vi "Create Asset.vi"(4 "Asset Class":enum16{"Undefined", "Asset", "Dut", "Fixture"}(ring), 5 "Vendor Number":u32, 6 "Bus Type":T1(ring), 7 "Vendor Name":string, 8 "Error In":errorcluster, 9 "Serial Number":string, 10 "Model Number":u32, 11 "Model Name":string) -> (0 "Error Out":errorcluster, 3 "Asset":refnum<class "Asset.lvclass">)   [LabVIEW 2019, in "Asset.lvclass"]
doc: "Creates an asset based on the properties that uniquely identify it."
uses:
  Asset.lvclass
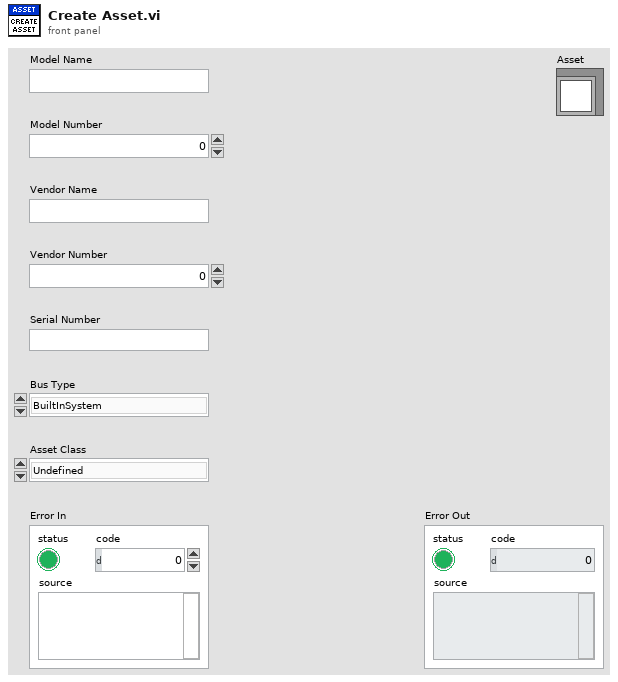
[diagram p1: front panel]
types:
  T1 = enum16{"BuiltInSystem", "PciPxi", "Usb", "Gpib", "Vxi", "Serial", "TcpIp", "cRio", "Scxi", "cDaq", "SwitchBlock", "Scc", "FireWire", "Accessory", "Can", "SwitchBlockDevice"}
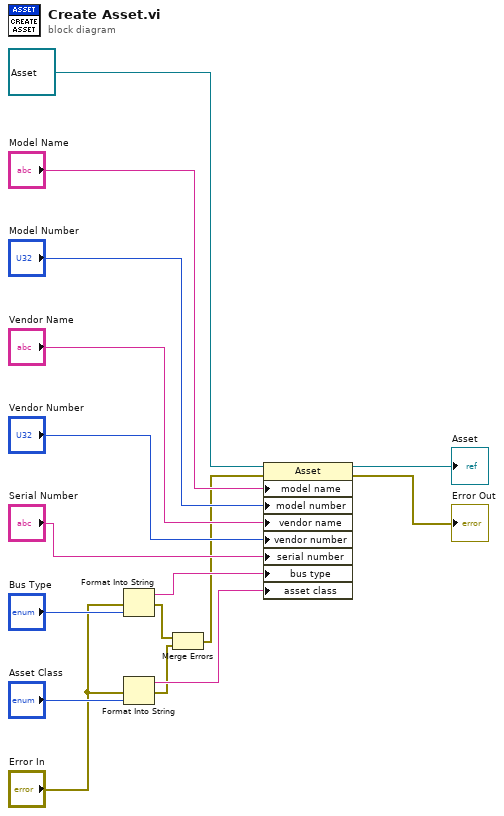
[diagram p0: block diagram]
diagram:
  n1 = Format Into String(error in="Error In", "Bus Type") -> (resulting string=w8:string, error out=w4:errorcluster)  [unwired: 2 in]
  n2 = Format Into String(error in="Error In", "Asset Class") -> (resulting string=w6:string, error out=w3:errorcluster)  [unwired: 2 in]
  n3 = Merge Errors(w4, w3) -> (w2:errorcluster)
  n4 = property class="Asset"(reference=refnum<class "Asset.lvclass"> refnum ("Asset.lvclass"), error in=w2, "model name"="Model Name", "model number"="Model Number", "vendor name"="Vendor Name", "vendor number"="Vendor Number", "serial number"="Serial Number", "bus type"=w8, "asset class"=w6) -> (reference out=→"Asset":refnum<class "Asset.lvclass">, error out=→"Error Out":errorcluster)
